vi "DSF.Engine.Framework.Set Hardware Info.vi"(10 "Hardware Info":refnum<class "DSF.Engine.Hardware Info.lvclass">, 11 "Framework in":refnum<class "DSF.Engine.Framework.lvclass">) -> (3 "Framework out":refnum<class "DSF.Engine.Framework.lvclass">)   [LabVIEW 2017, in "Data Sharing Framework Engine.lvlib" / "DSF.Engine.Framework.lvclass"]
uses:
  DSF.Engine.Framework.lvclass
  Hardware/DSF.Engine.Hardware Info.lvclass
  DSF.Engine.Framework.lvclass/DSF.Engine.Framework.ctl
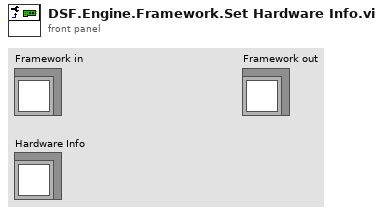
[diagram p1: front panel]
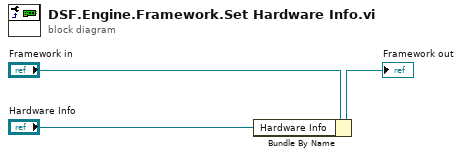
[diagram p0: block diagram]
diagram:
  n1 = Bundle By Name(cluster="Framework in", "Hardware Info"="Hardware Info") -> (→"Framework out":refnum<class "DSF.Engine.Framework.lvclass">)
